vi "Ramp&Triangle Waveform Generation.vi"(4 "Column":i32, 5 "File Name":string, 6 "#Bytes":u8, 7 "Step":sgl, 8 "error in":errorcluster, 9 "Max":sgl, 10 "Min":sgl, 11 "Type":string) -> (0 "error out":errorcluster, 3 "Pattern":u8[][](array[numeric]))   [LabVIEW 2018]
doc: "All Rights Reserved © 2017 SyncSols"
uses:
  <vilib>/Analysis/1siggen.llb/Ramp Pattern by Delta.vi
  <vilib>/Analysis/NI_AALBase.lvlib
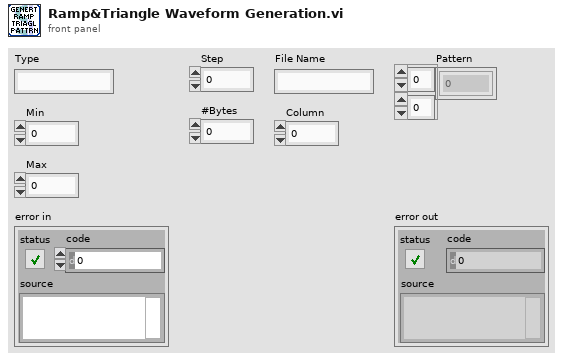
[diagram p1: front panel]
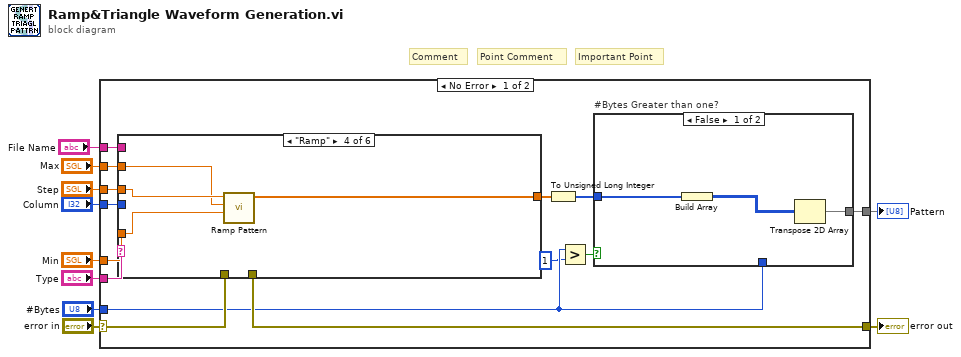
[diagram p0: block diagram]
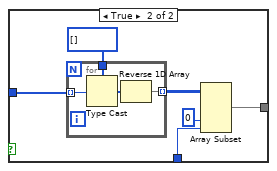
[diagram p2: hidden frame]
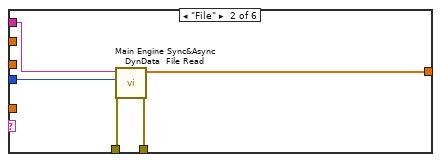
[diagram p4: hidden frame]
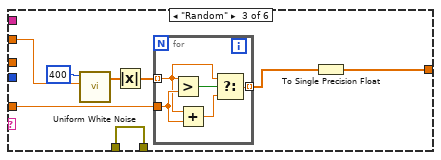
[diagram p5: hidden frame]
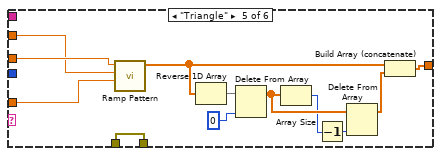
[diagram p6: hidden frame]
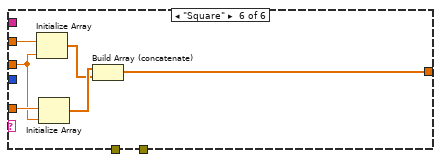
[diagram p7: hidden frame]
diagram:
  # "Important Point"
  # "Point Comment"
  # "Comment"
  n1 = case shown="No Error" "error in" {
    selector: "error in" -> [w18 w79]
    tunnel: [w17 w79] -> w10
    tunnel: "Type" -> [w24 _]
    tunnel: "Max" -> [w23 _]
    tunnel: "Step" -> [w21 _]
    tunnel: "Min" -> [w22 _]
    tunnel: [w20 _] -> w3
    tunnel: "#Bytes" -> [w14 _]
    tunnel: "File Name" -> [w16 _]
    tunnel: "Column" -> [w15 _]
    frame No Error {
      n2 = case shown="\"Ramp\"" w24 {
        tunnel: w23 -> [_ _ w49 w59 w66 w78]
        tunnel: w21 -> [_ _ _ w60 w68 w73]
        tunnel: w22 -> [_ _ w51 w58 w67 w77]
        tunnel: [_ w39 w45 w57 w71 w74] -> w19
        tunnel: w18 -> [w38 w42 w44 _ w70 _]
        tunnel: [w38 w43 w44 _ w70 _] -> w17
        tunnel: w16 -> [_ w41 _ _ _ _]
        tunnel: w15 -> [_ w40 _ _ _ _]
        frame Default {
        }
        frame "File" {
          n3 = call "Main Engine Sync&Async DynData  File Read.vi"("error in"=w42, "Column"=w40, "File Name"=w41) -> ("error out"=w43:errorcluster, "File DynData"=w39:sgl[])  [unwired: 7 in]
        }
        frame "Random" {
          n4 = call <vilib>:"Uniform White Noise.vi"("amplitude"=w49, "samples"=400) -> ("uniform white noise"=w48:dbl[])  [unwired: 8 in, 1 out]
          n5 = Absolute Value(x=w48) -> (abs(x)=w47:dbl[])
          n6 = for {
            tunnel: w51 -> [w55]
            tunnel: w47 -> [w54] mode=indexing
            tunnel: [w52] -> w46 mode=indexing
            n7 = Greater?(x=w54, y=w55) -> (0:w56:bool)
            n8 = Add(x=w54, y=w55) -> (x+y=w53:dbl)
            n9 = Select(t=w54, s=w56, f=w53) -> (s? t:f=w52:dbl)
          }
          n10 = To Single Precision Float(number=w46) -> (single precision float=w45:sgl[])
        }
        frame "Ramp" {
          n11 = call-poly <vilib>:"Ramp Pattern.vi"("start"=w58, "end"=w59, "delta"=w60) -> ("Ramp Pattern"=w57:dbl[])  [unwired: 6 in, 2 out]
        }
        frame "Triangle" {
          n12 = call-poly <vilib>:"Ramp Pattern.vi"("start"=w67, "end"=w66, "delta"=w68) -> ("Ramp Pattern"=w65:dbl[])  [unwired: 6 in, 2 out]
          n13 = Reverse 1D Array(array=w65) -> (reversed array=w72:dbl[])
          n14 = Delete From Array(array=w72, index=0) -> (array with subset deleted=w64:dbl[])  [unwired: 1 in, 1 out]
          n15 = Array Size(array=w64) -> (size(s)=w62:i32)
          n16 = Decrement(x=w62) -> (x-1=w63:i32)
          n17 = Delete From Array(array=w64, index=w63) -> (array with subset deleted=w61:dbl[])  [unwired: 1 in, 1 out]
          n18 = Build Array (concatenate)(w65, w61) -> (w71:dbl[])
        }
        frame "Square" {
          n19 = Initialize Array(w78, w73) -> (w75:sgl[])
          n20 = Initialize Array(w77, w73) -> (w76:sgl[])
          n21 = Build Array (concatenate)(w76, w75) -> (w74:sgl[])
        }
      }
      n22 = To Unsigned Long Integer(number=w19) -> (unsigned 32bit integer=w11:u32[])
      n23 = Greater?(x=w14, y=u8 1) -> (0:w12:bool)
      n24 = case "#Bytes Greater than one?" shown="False" w12 {
        tunnel: [w25 w30] -> w20
        tunnel: w11 -> [w27 w28]
        tunnel: w14 -> [_ w31]
        frame False {
          n25 = Build Array(w27) -> (w26:u32[][])
          n26 = Transpose 2D Array(2D array=w26) -> (transposed array=w25:u32[][])
        }
        frame True {
          n27 = for {
            tunnel: w28 -> [w36] mode=indexing
            tunnel: u8[] [] -> [w37]
            tunnel: [w34] -> w32 mode=indexing
            n28 = Type Cast(type=w37, x=w36) -> (*(type *) &x=w35:u8[])
            n29 = Reverse 1D Array(array=w35) -> (reversed array=w34:u8[])
          }
          n30 = Array Subset(array=w32, index (col)=0 ("index"), length (col)=w31) -> (w30:u8[][])  [unwired: 2 in]
        }
      }
    }
    frame Error {
    }
  }
  "error out" <- w10
  "Pattern" <- w3
